vi "1_CalibrateCameraHeight.vi"(0 "Inputs: Collect Images":T5={"Image feed"=refnum, "Axes Speeds [mm/s]"={"X Speed"=10.0, "Y Speed"=10.0, "Z Speed"=10.0}, "XYZ .NET Refnum in"=refnum}, 1 "Current Build Phase":refnum<vi>, 2 "Autofocus Coordinates":T1, 3 "Focusing test range [mm]":dbl, 4 "Stepsize [mm]":dbl, 5 "error in (no error)":errorcluster, 6 "Templates directory":path, 7 "Time & Temperature Stamp":dbl[](array[numeric]), 8 "Path to save collected images":path=path "E:/XYZstage+Camera_CollectedImages/12-17-2016/images", 9 "milliseconds to wait":u32=3500) -> (14 "Optimized working distance [mm]":dbl, 15 "Uncertainty on optimized Z [mm]":dbl, 16 "Outputs: Collect Images":T3, 19 "error out":errorcluster)   [LabVIEW 2016]
uses:
  C:/Users/Aerotech/Documents/BNLStaveAssembly-blueprint/Bin/Aerotech.A3200.dll
  BNLStaveAssembly-blueprint/Bin/Aerotech.A3200.dll
panel:
  in  "Tab Control":enum32{"Inputs", "Results", "Error handling"}(tab)
  out "Radius vs Height: Linear Fit Results":T2
  # "CALIBRATE CAMERA HEIGHT Brandeis University - Brookhaven National Laboratory * ATLAS Phase II Inner Tracker Upgrade"
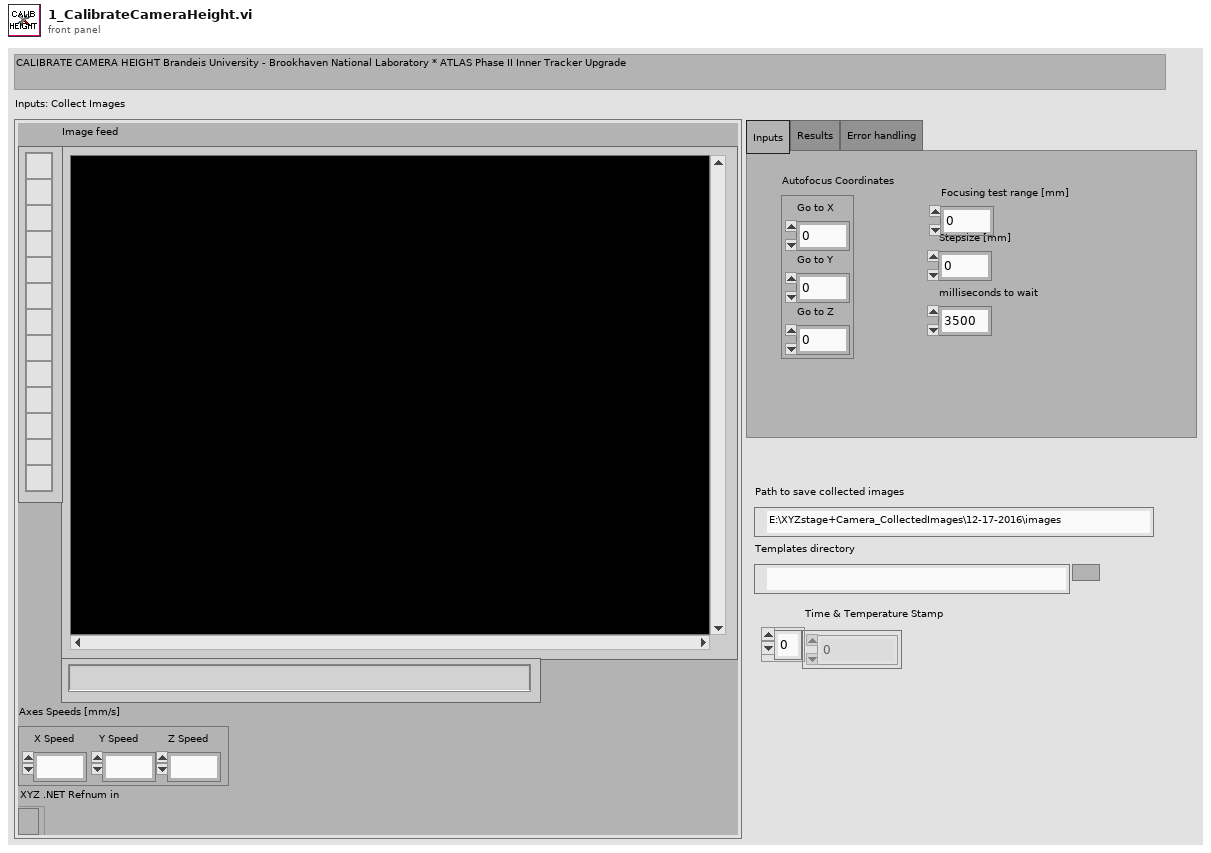
[diagram p1: front panel]
types:
  T1 = cluster{"Go to X":dbl, "Go to Y":dbl, "Go to Z":dbl}
  T2 = cluster{"Slope":dbl, "Slope uncertainty":dbl, "Intercept":dbl, "Intercept uncertainty":dbl}
  T3 = cluster{"Captured positions":dbl[][], "XYZ .NET Refnum out":refnum<k24>}
  T4 = typedef "IMAQ Image.ctl" = refnum<image>
  T5 = cluster{"Image feed":T4, "Axes Speeds [mm/s]":cluster{"X Speed":dbl, "Y Speed":dbl, "Z Speed":dbl}, "XYZ .NET Refnum in":refnum<k24>}
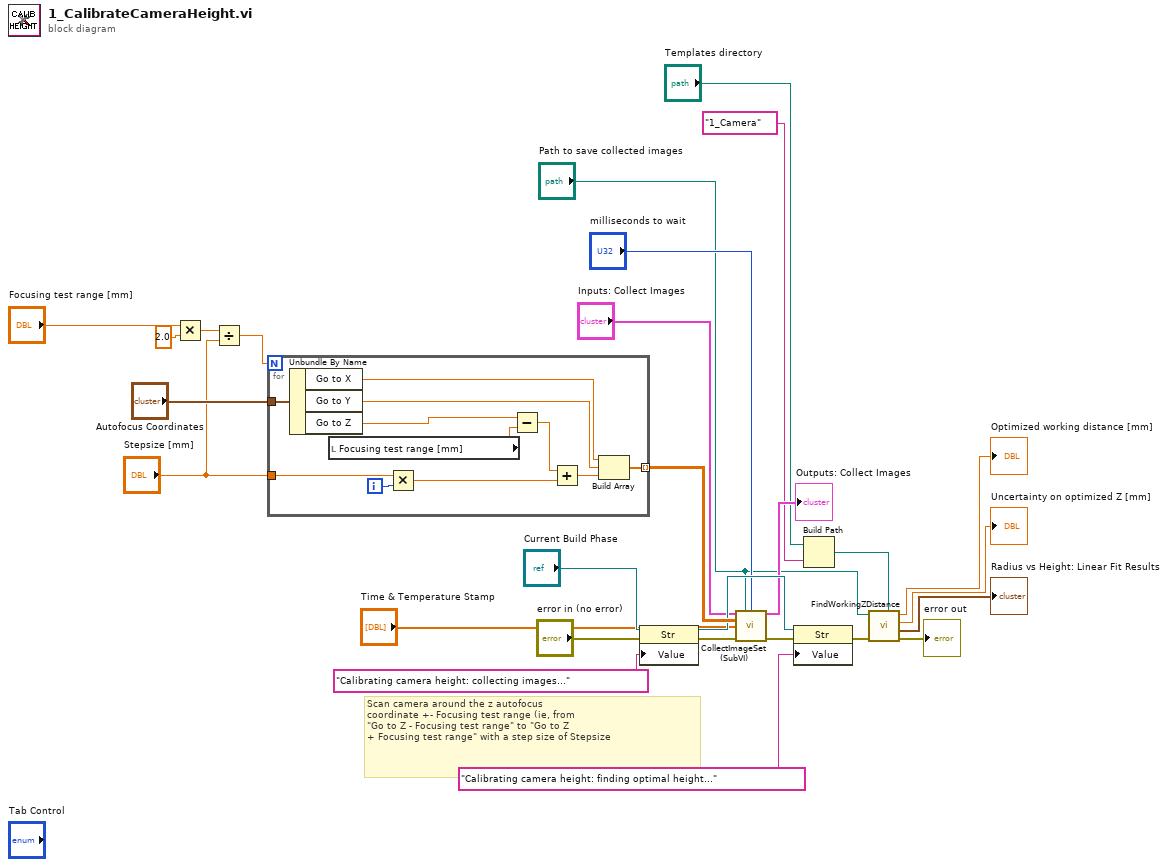
[diagram p0: block diagram]
diagram:
  # "Scan camera around the z autofocus\ncoordinate +- Focusing test range (ie, from\n\"Go to Z - Focusing test range\" to \"Go to Z \n+ Focusing test range\" with a step size of Stepsize"
  n1 = Multiply(x="Focusing test range [mm]", y=2.0) -> (x*y=w22:dbl)
  n2 = Divide(x=w22, y="Stepsize [mm]") -> (x/y=w24:dbl)
  n3 = for {
    N: w24 -> [_]
    tunnel: "Autofocus Coordinates" -> [w38]
    tunnel: [w35] -> w26 mode=indexing
    tunnel: "Stepsize [mm]" -> [w33]
    i -> [w34]
    n4 = Unbundle By Name(w38) -> ("Go to X"=w37:dbl, "Go to Y"=w36:dbl, "Go to Z"=w32:dbl)
    n5 = local read "Focusing test range [mm]"() -> (w31:dbl)
    n6 = Multiply(x=w33, y=w34) -> (x*y=w29:dbl)
    n7 = Subtract(x=w32, y=w31) -> (x-y=w30:dbl)
    n8 = Add(x=w30, y=w29) -> (x+y=w28:dbl)
    n9 = Build Array(w37, w36, w28) -> (w35:dbl[])
  }
  n10 = property class="Str"(reference="Current Build Phase", error in="error in (no error)", "Value"="Calibrating camera height: collecting images...") -> (reference out=w19:refnum<vi>, error out=w13:errorcluster)
  n11 = call "CollectImageSet (SubVI).vi"("Inputs"="Inputs: Collect Images", "Path to save collected images"="Path to save collected images", "milliseconds to wait"="milliseconds to wait", "Set of coordinates to process"=w26, "Time & Temperature Stamp"="Time & Temperature Stamp", "error in"=w13) -> ("Outputs"=→"Outputs: Collect Images":T3, "error out"=w20:errorcluster)  [unwired: 7 in, 1 out]
  n12 = property class="Str"(reference=w19, error in=w20, "Value"="Calibrating camera height: finding optimal height...") -> (error out=w4:errorcluster)  [unwired: 1 out]
  n13 = Build Path(base path="Templates directory", name or relative path="1_Camera") -> (appended path=w5:path)
  n14 = call "FindWorkingZDistance.vi"("Template File Path"=w5, "error in"=w4, "Images Directory"="Path to save collected images") -> ("error out"=→"error out":errorcluster, "Radius vs Height: Linear Fit Results"=→"Radius vs Height: Linear Fit Results":T2, "Uncertainty on optimized Z"=→"Uncertainty on optimized Z [mm]":dbl, "Optimized Z"=→"Optimized working distance [mm]":dbl)  [unwired: 5 in]
